vi "Robot Main.vi"() -> ()   [LabVIEW 2015]
doc: "This VI implements the framework and scheduler for your robotics program. It should not be necessary to modify the framework. You are expected to add your code to the VIs called from Robot Main - the ones located in the Team Code folder within the project."
uses:
  <vilib>/Rock Robotics/WPI/Camera/WPI_CameraImageSize.ctl
  Team Code/Robot Global Data.vi
panel:
  in  "stop":bool
  in  "Image Size":T1=enum."320x240"
  in  "Finish":bool
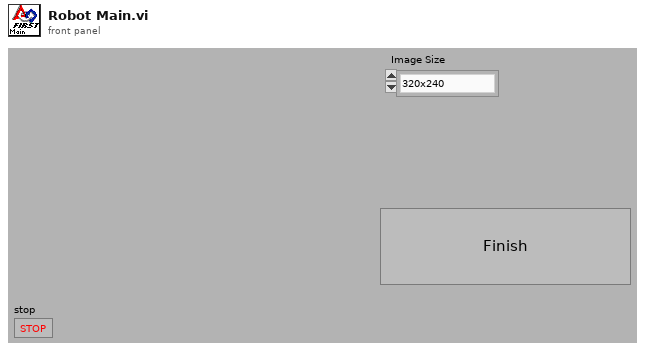
[diagram p1: front panel]
types:
  T1 = typedef "WPI_CameraImageSize.ctl" = enum16{"640x480", "320x240", "160x120", "Custom"}
  T2 = typedef "WPI_DriverStationMatch Info.ctl" = cluster{"Autonomous Elapsed Seconds":dbl, "TeleOp Elapsed Seconds":dbl, "Disabled Elapsed Seconds":dbl, "Visited Autonomous":bool, "Visited TeleOp":bool, "Visited Disabled":bool, "Autonomous Settings":cluster{"Autonomous Style":enum16{"Iterative", "Independent"}, "VI Refnum":refnum<vi>}}
  T3 = typedef "WPI_DriverStationDerivedRobotMode.ctl" = enum16{"Init", "Execute", "Stop"}
  T4 = typedef "WPI_DriverStationRobotMode2.ctl" = enum16{"Autonomous Disabled", "Autonomous Enabled", "Teleop Disabled", "Teleop Enabled", "Disconnected", "Finish", "Test Disabled", "Test Enabled", "Emergency Stopped"}
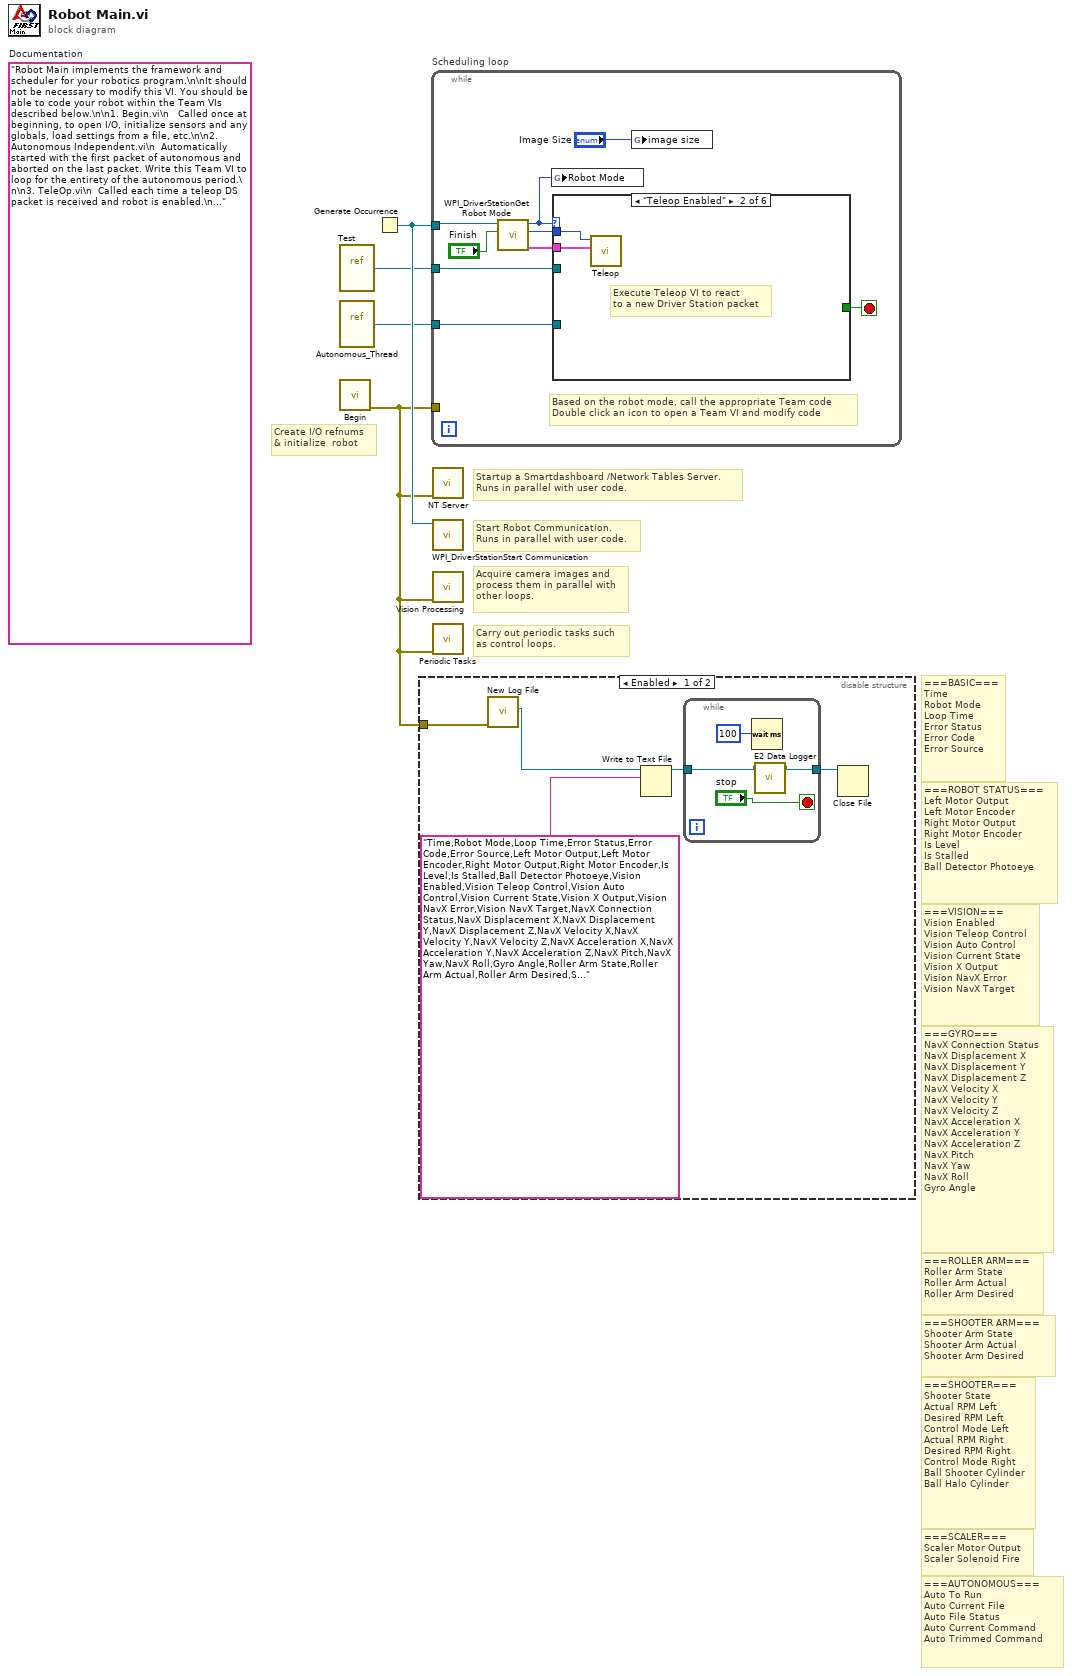
[diagram p0: block diagram]
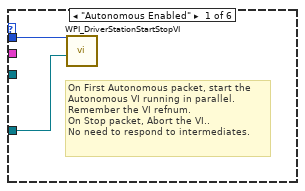
[diagram p3: hidden frame]
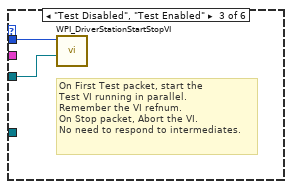
[diagram p4: hidden frame]
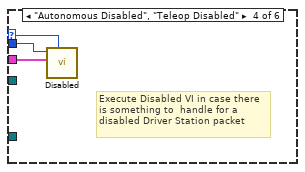
[diagram p5: hidden frame]
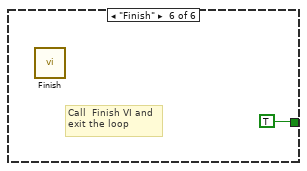
[diagram p7: hidden frame]
diagram:
  (unwired) "Robot Main implements the framework and scheduler for your robotics program.\n\nIt should not be necessary to modify this VI. You should be able to code your robot within the Team VIs described below.\n\n1. Begin.vi\n   Called once at beginning, to open I/O, initialize sensors and any globals, load settings from a file, etc.\n\n2. Autonomous Independent.vi\n  Automatically started with the first packet of autonomous and aborted on the last packet. Write this Team VI to loop for the entirety of the autonomous period.\n\n3. TeleOp.vi\n  Called each time a teleop DS packet is received and robot is enabled.\n\n4. Disabled.vi\n  Called each time a packet is received and the robot is disabled.\n\n5. Test.vi\n  Called Automatically started with the first test packet and aborted on the last. Modify this VI to carry out robot and sensor validation tests.\n\n6. Vision.vi\n  A parallel loop that acquires and processes camera images.\n\n7. PeriodicTasks.vi\n  Parallel loops running at user-defined rates.\n\n8. Finish.vi\n  Called before exiting, so you can save data, clean up I/O, etc.\n"  # Documentation
  # "===SCALER===\nScaler Motor Output\nScaler Solenoid Fire"
  # "===VISION===\nVision Enabled\nVision Teleop Control\nVision Auto Control\nVision Current State\nVision X Output\nVision NavX Error\nVision NavX Target"
  # "===SHOOTER ARM===\nShooter Arm State\nShooter Arm Actual\nShooter Arm Desired"
  # "===ROLLER ARM===\nRoller Arm State\nRoller Arm Actual\nRoller Arm Desired"
  # "===ROBOT STATUS===\nLeft Motor Output\nLeft Motor Encoder\nRight Motor Output\nRight Motor Encoder\nIs Level\nIs Stalled\nBall Detector Photoeye"
  # "===AUTONOMOUS===\nAuto To Run\nAuto Current File\nAuto File Status\nAuto Current Command\nAuto Trimmed Command"
  # "===SHOOTER===\nShooter State\nActual RPM Left\nDesired RPM Left\nControl Mode Left\nActual RPM Right\nDesired RPM Right\nControl Mode Right\nBall Shooter Cylinder\nBall Halo Cylinder"
  # "===BASIC===\nTime \nRobot Mode\nLoop Time\nError Status\nError Code\nError Source"
  # "===GYRO===\nNavX Connection Status\nNavX Displacement X\nNavX Displacement Y\nNavX Displacement Z\nNavX Velocity X\nNavX Velocity Y\nNavX Velocity Z\nNavX Acceleration X\nNavX Acceleration Y\nNavX Acceleration Z\nNavX Pitch\nNavX Yaw\nNavX Roll\nGyro Angle"
  # "Startup a Smartdashboard /Network Tables Server.\nRuns in parallel with user code."
  # "Carry out periodic tasks such\nas control loops."
  # "Acquire camera images and\nprocess them in parallel with\nother loops."
  # "Create I/O refnums\n& initialize  robot"
  # "Start Robot Communication.\nRuns in parallel with user code."
  n1 = vi-ref "Test.vi"() -> (w2:refnum<vi>)
  n2 = vi-ref "Autonomous_Thread.vi"() -> (w3:refnum<vi>)
  n3 = call "Begin.vi"() -> ("error out"=w1:errorcluster)  [unwired: 2 in, 9 out]
  n4 = Generate Occurrence() -> (w4:refnum<k4>)
  n5 = disable-structure shown="Enabled" {
    disable-tunnel: w1 -> [w5 _]
    frame Enabled {
      n6 = call "New Log File.vi"("error in (no error)"=w5) -> ("refnum out"=w6:refnum<file>)  [unwired: 9 in]
      n7 = Write to Text File(file (use dialog)=w6, text="Time,Robot Mode,Loop Time,Error Status,Error Code,Error Source,Left Motor Output,Left Motor Encoder,Right Motor Output,Right Motor Encoder,Is Level,Is Stalled,Ball Detector Photoeye,Vision Enabled,Vision Teleop Control,Vision Auto Control,Vision Current State,Vision X Output,Vision NavX Error,Vision NavX Target,NavX Connection Status,NavX Displacement X,NavX Displacement Y,NavX Displacement Z,NavX Velocity X,NavX Velocity Y,NavX Velocity Z,NavX Acceleration X,NavX Acceleration Y,NavX Acceleration Z,NavX Pitch,NavX Yaw,NavX Roll,Gyro Angle,Roller Arm State,Roller Arm Actual,Roller Arm Desired,Shooter Arm State,Shooter Arm Actual,Shooter Arm Desired,Shooter State,Actual RPM Left,Desired RPM Left,Control Mode Left,Actual RPM Right,Desired RPM Right,Control Mode Right,Ball Shooter Cylinder,Ball Halo Cylinder,Scaler Motor Output,Scaler Solenoid Fire,Auto To Run,Auto Current File,Auto File Status,Auto Current Command,Auto Trimmed Command,Shooter Amps Left,Shooter Amps Right, Vision After Offset") -> (refnum out=w9:refnum<file>)  [unwired: 1 in, 3 out]
      n8 = while {
        tunnel: w9 -> [w11]
        tunnel: [w10] -> w8
        stop <- "stop" stop-if-true
        n9 = Wait (ms)(milliseconds to wait=u32 100 ("millisecond multiple")) -> ()  [unwired: 1 out]
        n10 = call "E2 Data Logger.vi"("refnum in"=w11) -> ("refnum out"=w10:refnum<file>)  [unwired: 6 in]
      }
      n11 = Close File(refnum=w8) -> ()  [unwired: 1 in, 2 out]
    }
    frame Disabled {
    }
  }
  n12 = while "Scheduling loop" {
    tunnel: w4 -> [w21]
    tunnel: w1 -> [_]
    tunnel: w3 -> [w17]
    tunnel: w2 -> [w15]
    stop <- w18 stop-if-true
    # "Based on the robot mode, call the appropriate Team code\nDouble click an icon to open a Team VI and modify code"
    n13 = call <vilib>:"WPI_DriverStationGet Robot Mode.vi"("Finish"="Finish", "DS Occurrence"=w21) -> ("Match Info out"=w19:T2, "Call Context"=w22:T3, "Robot Mode"=w14:T4)  [unwired: 7 out]
    n14 = global write "Robot Global Data.vi" "Robot Mode"(w14) -> ()
    n15 = case shown="\"Teleop Enabled\"" w14 {
      selector: w14 -> [_ _ _ w29 _ _]
      tunnel: w22 -> [w24 w26 w28 w31 _ _]
      tunnel: w19 -> [_ w25 _ w30 _ _]
      tunnel: [_ _ _ _ _ TRUE] -> w18
      tunnel: w17 -> [w23 _ _ _ _ _]
      tunnel: w15 -> [_ _ w27 _ _ _]
      frame "Autonomous Enabled" {
        # "On First Autonomous packet, start the\nAutonomous VI running in parallel.\nRemember the VI refnum.\nOn Stop packet, Abort the VI..\nNo need to respond to intermediates."
        n16 = call <vilib>:"WPI_DriverStationStartStopVI.vi"("VI in"=w23, "Call Context"=w24) -> ()  [unwired: 10 in]
      }
      frame "Teleop Enabled" {
        # "Execute Teleop VI to react\nto a new Driver Station packet"
        n17 = call "Teleop.vi"("Match Info"=w25, "Call Context"=w26) -> ()  [unwired: 1 in, 9 out]
      }
      frame "Test Disabled", "Test Enabled" {
        # "On First Test packet, start the\nTest VI running in parallel.\nRemember the VI refnum.\nOn Stop packet, Abort the VI.\nNo need to respond to intermediates."
        n18 = call <vilib>:"WPI_DriverStationStartStopVI.vi"("VI in"=w27, "Call Context"=w28) -> ()  [unwired: 10 in]
      }
      frame "Autonomous Disabled", "Teleop Disabled" {
        # "Execute Disabled VI in case there\nis something to  handle for a\ndisabled Driver Station packet"
        n19 = call "Disabled.vi"("Robot Mode"=w29, "Match Info"=w30, "Call Context"=w31) -> ()  [unwired: 1 in, 8 out]
      }
      frame "Disconnected", Default {
        # "Driver Station packet didn't arrive.\nPossibly useful for diagnostics"
      }
      frame "Finish" {
        # "Call  Finish VI and\nexit the loop"
        n20 = call "Finish.vi"() -> ()  [unwired: 1 in, 7 out]
      }
    }
    n21 = global write "Robot Global Data.vi" "image size"("Image Size") -> ()
  }
  n22 = call <vilib>:"NT Server.vi"("error in (no error)"=w1) -> ()  [unwired: 11 in]
  n23 = call <vilib>:"WPI_DriverStationStart Communication.vi"("occurrence"=w4) -> ()  [unwired: 1 in, 10 out]
  n24 = call "Vision Processing.vi"("error in (no error)"=w1) -> ()  [unwired: 1 in, 6 out]
  n25 = call "Periodic Tasks.vi"("error in"=w1) -> ()  [unwired: 1 in, 10 out]
